vi "Cycle 4 Main Spin.vi"(0 "GEA2 Reference In":refnum<k24>, 1 "Basket Speeds (rpm)":u32[](array[numeric])=[125, 450, 700], 5 "GEA Inputs":T1={"Source"=228, "Destination"=35} {"Destination" format="%.0x"; "Source" format="%.0x"}, 7 "Standalone?":bool, 9 "Dwell Times (s)":dbl[](array[numeric])=[90.0, 30.0, 600.0], 11 "Error In":errorcluster, 12 "Basket Speed Tolerance (rpm)":u32=2) -> (4 "GEA2 Reference Out":refnum<k24>, 6 "Pass/Fail?":bool, 8 "Report Text":string, 15 "Error Out":errorcluster)   [LabVIEW 2016, in "2015 VA Washer.lvlib"]
uses:
  Projects/2015 VA Washer.lvlib
  C:/Automation/DLLs/PC Dot Net/GeaCommunication.dll
  Common/LabVIEW GEA2 Toolkit/LabVIEW_GEA2_Toolkit.lvlibp/type defs/Source_Destination.ctl
  Common/LabVIEW GEA2 Toolkit/LabVIEW_GEA2_Toolkit.lvlibp/type defs/ERD Read Data In.ctl
  Common/LabVIEW GEA2 Toolkit/LabVIEW_GEA2_Toolkit.lvlibp/type defs/Data Type.ctl
  Valew Common/type defs/Drive Cycle Engine Request State.ctl
  Common/LabVIEW GEA2 Toolkit/LabVIEW_GEA2_Toolkit.lvlibp
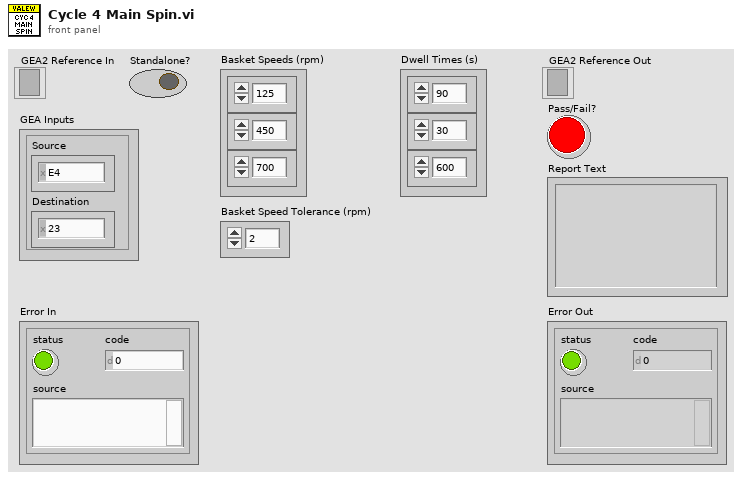
[diagram p1: front panel]
types:
  T1 = typedef "LabVIEW_GEA2_Toolkit.lvlibp/Source_Destination.ctl" = cluster{"Source":u8, "Destination":u8}
  T2 = typedef "2015 VA Washer.lvlib/Drive Cycle Engine Request State.ctl" = enum16{"Start", "Stop", "Pause", "Resume", "Select"}
  T3 = typedef "LabVIEW_GEA2_Toolkit.lvlibp/ERD Read Data In.ctl" = cluster{"ERD Number":u16, "Data Type":T4}
  T4 = typedef "LabVIEW_GEA2_Toolkit.lvlibp/Data Type.ctl" = enum16{"string", "boolean", "uint8_t", "uint16_t", "uint32_t", "uint64_t", "int8_t", "int16_t", "int32_t", "int64_t"}
  T5 = typedef "LabVIEW_GEA2_Toolkit.lvlibp/ERD Read Data Out.ctl" = cluster{"ERD Number":u16, "Data":string}
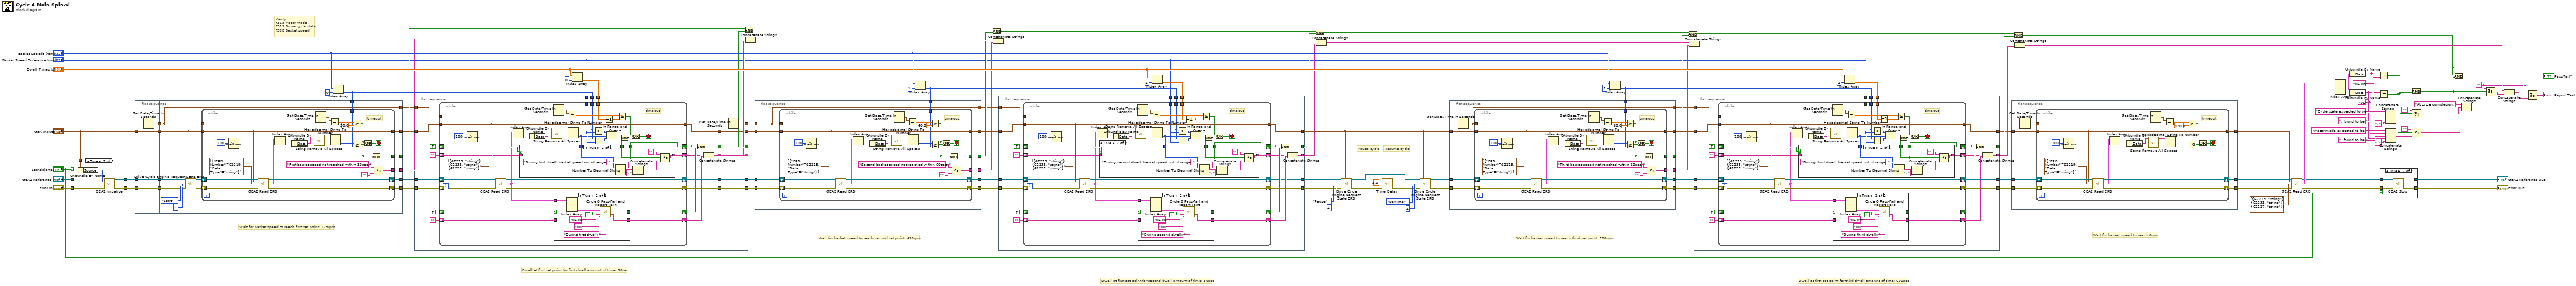
[diagram p0: block diagram]
diagram:
  w9 = ""
  w116 = "04 0B" ("y")
  w104 = "06" ("y")
  # "Wait for basket speed to reach 0rpm"
  # "Resume cycle"
  # "Pause cycle"
  # "Dwell at first set point for third dwell amount of time: 600sec"
  # "Wait for basket speed to reach third set point: 700rpm"
  # "Dwell at first set point for second dwell amount of time: 30sec"
  # "Wait for basket speed to reach second set point: 450rpm"
  # "Verify\nF313 Motor mode\nF319 Drive cycle state\nF30B Basket speed"
  # "Dwell at first set point for first dwell amount of time: 90sec"
  # "Wait for basket speed to reach first set point: 125rpm"
  n1 = case shown="True" "Standalone?" {
    tunnel: "GEA2 Reference In" -> [w123 _]
    tunnel: [w123 w128] -> w25
    tunnel: "Error In" -> [w122 w127]
    tunnel: [w122 w126] -> w26
    tunnel: "GEA Inputs" -> [_ w125]
    frame False {
    }
    frame True {
      n2 = Unbundle By Name(w125) -> ("Source"=w124:u8)
      n3 = call "GEA2 Initialize.vi"("Source Address"=w124, "error in"=w127) -> ("GEA2 Reference Out"=w128:refnum<k24>, "error out"=w126:errorcluster)  [unwired: 11 in, 1 out]
    }
  }
  n4 = flat-sequence {
    tunnel: "GEA Inputs" -> [w132]
    tunnel: [w132] -> w27
    tunnel: w26 -> [w129]
    tunnel: w25 -> [w130]
    tunnel: [w131] -> w24
    tunnel: [w130] -> w23
    tunnel: [w129] -> w22
    tunnel: [w146] -> w84
    tunnel: [w145] -> w85
    tunnel: [w144] -> w97
    tunnel: [w141] -> w50
    tunnel: [w142] -> w48
    tunnel: w66 -> [w143]
    tunnel: [w133] -> w30
    tunnel: w27 -> [w134]
    tunnel: w24 -> [w133]
    tunnel: w23 -> [w138]
    tunnel: w22 -> [w137]
    frame #0 {
      n5 = Get Date/Time In Seconds() -> (seconds since 1Jan1904=w131:timestamp)
    }
    frame #1 {
      n6 = call "Drive Cycle Engine Request State ERD.vi"("GEA2 Reference In"=w138, "GEA Inputs"=w134, "Cycle ID"=u8 4, "Drive Cycle Engine Request State"=Drive_Cycle_Engine_Request_State."Start", "Error In"=w137) -> ("GEA2 Reference Out"=w136:refnum<k24>, "Error Out"=w135:errorcluster)  [unwired: 9 in]
      n7 = while {
        shift-right: [w169] -> w146
        shift-left: w135 -> [w170]
        shift-right: [w167] -> w145
        shift-left: w136 -> [w168]
        tunnel: w134 -> [w165]
        tunnel: [w165] -> w144
        tunnel: w133 -> [w147]
        tunnel: w143 -> [w155]
        tunnel: [w150] -> w142
        tunnel: [w148] -> w141
        stop <- w162 stop-if-true
        # "timeout"
        n8 = Wait (ms)(milliseconds to wait=u32 100) -> ()  [unwired: 1 out]
        n9 = call "GEA2 Read ERD.vi"("GEA2 Reference In"=w168, "GEA Inputs"=w165, "Read ERD List"=T3[] [{"ERD Number"=62219, "Data Type"=enum."string"}], "Error In"=w170) -> ("GEA2 Reference Out"=w167:refnum<k24>, "ERD Data Out"=w154:T5[], "Error Out"=w169:errorcluster)  [unwired: 8 in, 1 out]
        n10 = Index Array(array=w154) -> (element=w166:T5)  [unwired: 1 in]
        n11 = Unbundle By Name(w166) -> ("Data"=w158:string)
        n12 = call "String Remove All Spaces.vi"("Input String"=w158) -> ("Spaces Removed"=w159:string)  [unwired: 13 in, 1 out]
        n13 = Get Date/Time In Seconds() -> (seconds since 1Jan1904=w163:timestamp)
        n14 = Subtract(x=w163, y=w147) -> (x-y=w164:dbl)
        n15 = Hexadecimal String To Number(string=w159) -> (number=w157:u32)  [unwired: 2 in, 1 out]
        n16 = Greater Or Equal?(x=w164, y=30.0) -> (x >= y?=w149:bool)
        n17 = Greater Or Equal?(x=w157, y=w155) -> (x >= y?=w153:bool)
        n18 = Or(x=w149, y=w153) -> (x .or. y?=w162:bool)
        n19 = Not(x=w149) -> (.not. x?=w148:bool)
        n20 = Select(t="First basket speed not reached within 30sec. ", s=w149, f="") -> (s? t:f=w150:string)
      }
    }
  }
  n21 = Index Array(array="Basket Speeds (rpm)", index=0) -> (element=w66:u32)
  n22 = flat-sequence {
    tunnel: w87 -> [w183]
    tunnel: w66 -> [w182]
    tunnel: "Basket Speed Tolerance (rpm)" -> [w181]
    tunnel: w84 -> [w188]
    tunnel: w97 -> [w189]
    tunnel: w85 -> [w190]
    tunnel: w30 -> [w171]
    tunnel: [w186] -> w5
    tunnel: [w185] -> w4
    tunnel: [w184] -> w3
    tunnel: [w175] -> w2
    tunnel: [w172] -> w1
    tunnel: [w245] -> w6
    tunnel: [w246] -> w47
    tunnel: [w247] -> w49
    tunnel: [w248] -> w81
    tunnel: [w249] -> w83
    tunnel: [w250] -> w82
    tunnel: w5 -> [w250]
    tunnel: w4 -> [w249]
    tunnel: w3 -> [w248]
    tunnel: w2 -> [w247]
    tunnel: w1 -> [w246]
    frame #0 {
      n23 = while {
        shift-right: [w222] -> w186
        shift-left: w188 -> [w223]
        shift-right: [w220] -> w185
        shift-left: w190 -> [w221]
        tunnel: w189 -> [w218]
        tunnel: [w218] -> w184
        tunnel: w171 -> [w216]
        shift-right: [w200] -> w176
        shift-left: TRUE -> [w202]
        tunnel: w183 -> [w192]
        tunnel: w182 -> [w207]
        tunnel: w181 -> [w206]
        shift-right: [w204] -> w173
        shift-left: "" -> [w201]
        shift-right: [w194] -> w177
        shift-left: TRUE -> [w197]
        shift-right: [w195] -> w174
        shift-left: "" -> [w196]
        stop <- w214 stop-if-true
        # "timeout"
        n24 = Wait (ms)(milliseconds to wait=u32 100) -> ()  [unwired: 1 out]
        n25 = call "GEA2 Read ERD.vi"("GEA2 Reference In"=w221, "GEA Inputs"=w218, "Read ERD List"=T3[] [{"ERD Number"=62219, "Data Type"=enum."string"}, {"ERD Number"=62233, "Data Type"=enum."string"}, {"ERD Number"=62227, "Data Type"=enum."string"}], "Error In"=w223) -> ("GEA2 Reference Out"=w220:refnum<k24>, "ERD Data Out"=w193:T5[], "Error Out"=w222:errorcluster)  [unwired: 8 in, 1 out]
        n26 = Index Array(array=w193) -> (element=w219:T5)  [unwired: 1 in]
        n27 = Unbundle By Name(w219) -> ("Data"=w210:string)
        n28 = call "String Remove All Spaces.vi"("Input String"=w210) -> ("Spaces Removed"=w211:string)  [unwired: 13 in, 1 out]
        n29 = Get Date/Time In Seconds() -> (seconds since 1Jan1904=w215:timestamp)
        n30 = case shown="True" w197 {
          selector: w197 -> [w224 _]
          tunnel: w196 -> [w225 _]
          tunnel: [w225 w233] -> w195
          tunnel: [w224 w234] -> w194
          tunnel: w193 -> [_ w232]
          frame False {
          }
          frame True {
            n31 = Index Array(array=w232) -> (element #2=w230:T5, element #3=w229:T5)  [unwired: 3 in, 1 out]
            n32 = call "Cycle 0 Pass-Fail and Report Text.vi"("Drive Cycle State"=w230, "Motor Mode"=w229, "Previous Pass/Fail"=TRUE, "Cycle State Expected"="04 06", "Motor Mode Expected"="00", "Header"="During first dwell: ") -> ("Pass/Fail?"=w234:bool, "Report Text"=w233:string)  [unwired: 8 in]
          }
        }
        n33 = Subtract(x=w215, y=w216) -> (x-y=w217:dbl)
        n34 = Hexadecimal String To Number(string=w211) -> (number=w205:u32)  [unwired: 2 in, 1 out]
        n35 = Add(x=w207, y=w206) -> (x+y=w209:u32)
        n36 = Subtract(x=w207, y=w206) -> (x-y=w208:u32)
        n37 = Decrement(x=w192) -> (x-1=w191:dbl)
        n38 = In Range and Coerce(upper limit=w209, x=w205, lower limit=w208) -> (In Range?=w203:bool)  [unwired: 1 out]
        n39 = case shown="True" w202 {
          selector: w202 -> [w235 _]
          tunnel: w205 -> [_ w242]
          tunnel: [w236 w239] -> w204
          tunnel: w203 -> [_ w238]
          tunnel: w201 -> [w236 _]
          tunnel: [w235 w238] -> w200
          frame False {
          }
          frame True {
            n40 = Number To Decimal String(number=w242) -> (decimal integer string=w241:string)  [unwired: 1 in]
            n41 = Concatenate Strings("During first dwell, basket speed out of range: " ("string"), w241, ". " ("string")) -> (w240:string)
            n42 = Select(t="", s=w238, f=w240) -> (s? t:f=w239:string)
          }
        }
        n43 = Greater Or Equal?(x=w217, y=w191) -> (x >= y?=w198:bool)
        n44 = Not(x=w203) -> (.not. x?=w199:bool)
        n45 = Or(x=w198, y=w199) -> (x .or. y?=w214:bool)
      }
      n46 = And(x=w176, y=w177) -> (x .and. y?=w175:bool)
      n47 = Concatenate Strings(w173, w174) -> (w172:string)
    }
    frame #1 {
      n48 = Get Date/Time In Seconds() -> (seconds since 1Jan1904=w245:timestamp)
    }
  }
  n49 = Index Array(array="Dwell Times (s)", index=0) -> (element=w87:dbl)
  n50 = And(x=w50, y=w49) -> (x .and. y?=w46:bool)
  n51 = Concatenate Strings(w48, w47) -> (w45:string)
  n52 = flat-sequence {
    tunnel: [w257] -> w79
    tunnel: [w256] -> w78
    tunnel: [w255] -> w77
    tunnel: [w252] -> w43
    tunnel: [w253] -> w44
    tunnel: w76 -> [w254]
    tunnel: w82 -> [w258]
    tunnel: w81 -> [w259]
    tunnel: w83 -> [w260]
    tunnel: [w251] -> w29
    tunnel: w6 -> [w251]
    frame #0 {
      n53 = while {
        shift-right: [w283] -> w257
        shift-left: w258 -> [w284]
        shift-right: [w281] -> w256
        shift-left: w260 -> [w282]
        tunnel: w259 -> [w279]
        tunnel: [w279] -> w255
        tunnel: w251 -> [w261]
        tunnel: w254 -> [w269]
        tunnel: [w264] -> w253
        tunnel: [w262] -> w252
        stop <- w276 stop-if-true
        # "timeout"
        n54 = Wait (ms)(milliseconds to wait=u32 100) -> ()  [unwired: 1 out]
        n55 = call "GEA2 Read ERD.vi"("GEA2 Reference In"=w282, "GEA Inputs"=w279, "Read ERD List"=T3[] [{"ERD Number"=62219, "Data Type"=enum."string"}], "Error In"=w284) -> ("GEA2 Reference Out"=w281:refnum<k24>, "ERD Data Out"=w268:T5[], "Error Out"=w283:errorcluster)  [unwired: 8 in, 1 out]
        n56 = Index Array(array=w268) -> (element=w280:T5)  [unwired: 1 in]
        n57 = Unbundle By Name(w280) -> ("Data"=w272:string)
        n58 = call "String Remove All Spaces.vi"("Input String"=w272) -> ("Spaces Removed"=w273:string)  [unwired: 13 in, 1 out]
        n59 = Get Date/Time In Seconds() -> (seconds since 1Jan1904=w277:timestamp)
        n60 = Subtract(x=w277, y=w261) -> (x-y=w278:dbl)
        n61 = Hexadecimal String To Number(string=w273) -> (number=w271:u32)  [unwired: 2 in, 1 out]
        n62 = Greater Or Equal?(x=w278, y=60.0) -> (x >= y?=w263:bool)
        n63 = Greater Or Equal?(x=w271, y=w269) -> (x >= y?=w267:bool)
        n64 = Or(x=w263, y=w267) -> (x .or. y?=w276:bool)
        n65 = Not(x=w263) -> (.not. x?=w262:bool)
        n66 = Select(t="Second basket speed not reached within 60sec. ", s=w263, f="") -> (s? t:f=w264:string)
      }
    }
  }
  n67 = Index Array(array="Basket Speeds (rpm)", index=1) -> (element=w76:u32)
  n68 = And(x=w46, y=w43) -> (x .and. y?=w40:bool)
  n69 = Concatenate Strings(w45, w44) -> (w41:string)
  n70 = flat-sequence {
    tunnel: [w300] -> w60
    tunnel: [w299] -> w51
    tunnel: [w290] -> w39
    tunnel: [w287] -> w42
    tunnel: w74 -> [w298]
    tunnel: w76 -> [w297]
    tunnel: "Basket Speed Tolerance (rpm)" -> [w296]
    tunnel: w79 -> [w302]
    tunnel: w77 -> [w303]
    tunnel: w78 -> [w304]
    tunnel: [w286] -> w61
    tunnel: w29 -> [w285]
    frame #0 {
      n71 = while {
        shift-right: [w336] -> w300
        shift-left: w302 -> [w337]
        shift-right: [w334] -> w286
        shift-left: w304 -> [w335]
        tunnel: w303 -> [w332]
        tunnel: [w332] -> w299
        tunnel: w285 -> [w330]
        shift-right: [w314] -> w291
        shift-left: TRUE -> [w316]
        tunnel: w298 -> [w306]
        tunnel: w297 -> [w321]
        tunnel: w296 -> [w320]
        shift-right: [w318] -> w288
        shift-left: "" -> [w315]
        shift-right: [w308] -> w292
        shift-left: TRUE -> [w311]
        shift-right: [w309] -> w289
        shift-left: "" -> [w310]
        stop <- w328 stop-if-true
        # "timeout"
        n72 = Wait (ms)(milliseconds to wait=u32 100) -> ()  [unwired: 1 out]
        n73 = call "GEA2 Read ERD.vi"("GEA2 Reference In"=w335, "GEA Inputs"=w332, "Read ERD List"=T3[] [{"ERD Number"=62219, "Data Type"=enum."string"}, {"ERD Number"=62233, "Data Type"=enum."string"}, {"ERD Number"=62227, "Data Type"=enum."string"}], "Error In"=w337) -> ("GEA2 Reference Out"=w334:refnum<k24>, "ERD Data Out"=w307:T5[], "Error Out"=w336:errorcluster)  [unwired: 8 in, 1 out]
        n74 = Index Array(array=w307) -> (element=w333:T5)  [unwired: 1 in]
        n75 = Unbundle By Name(w333) -> ("Data"=w324:string)
        n76 = call "String Remove All Spaces.vi"("Input String"=w324) -> ("Spaces Removed"=w325:string)  [unwired: 13 in, 1 out]
        n77 = Get Date/Time In Seconds() -> (seconds since 1Jan1904=w329:timestamp)
        n78 = case shown="True" w311 {
          selector: w311 -> [w338 _]
          tunnel: w310 -> [w339 _]
          tunnel: [w339 w347] -> w309
          tunnel: [w338 w348] -> w308
          tunnel: w307 -> [_ w346]
          frame False {
          }
          frame True {
            n79 = Index Array(array=w346) -> (element #2=w344:T5, element #3=w343:T5)  [unwired: 3 in, 1 out]
            n80 = call "Cycle 0 Pass-Fail and Report Text.vi"("Drive Cycle State"=w344, "Motor Mode"=w343, "Previous Pass/Fail"=TRUE, "Cycle State Expected"="04 06", "Motor Mode Expected"="00", "Header"="During second dwell: ") -> ("Pass/Fail?"=w348:bool, "Report Text"=w347:string)  [unwired: 8 in]
          }
        }
        n81 = Subtract(x=w329, y=w330) -> (x-y=w331:dbl)
        n82 = Hexadecimal String To Number(string=w325) -> (number=w319:u32)  [unwired: 2 in, 1 out]
        n83 = Add(x=w321, y=w320) -> (x+y=w323:u32)
        n84 = Subtract(x=w321, y=w320) -> (x-y=w322:u32)
        n85 = Decrement(x=w306) -> (x-1=w305:dbl)
        n86 = In Range and Coerce(upper limit=w323, x=w319, lower limit=w322) -> (In Range?=w317:bool)  [unwired: 1 out]
        n87 = case shown="True" w316 {
          selector: w316 -> [w349 _]
          tunnel: w319 -> [_ w356]
          tunnel: [w350 w353] -> w318
          tunnel: w317 -> [_ w352]
          tunnel: w315 -> [w350 _]
          tunnel: [w349 w352] -> w314
          frame False {
          }
          frame True {
            n88 = Number To Decimal String(number=w356) -> (decimal integer string=w355:string)  [unwired: 1 in]
            n89 = Concatenate Strings("During second dwell, basket speed out of range: " ("string"), w355, ". " ("string")) -> (w354:string)
            n90 = Select(t="", s=w352, f=w354) -> (s? t:f=w353:string)
          }
        }
        n91 = Greater Or Equal?(x=w331, y=w305) -> (x >= y?=w312:bool)
        n92 = Not(x=w317) -> (.not. x?=w313:bool)
        n93 = Or(x=w312, y=w313) -> (x .or. y?=w328:bool)
      }
      n94 = And(x=w291, y=w292) -> (x .and. y?=w290:bool)
      n95 = Concatenate Strings(w288, w289) -> (w287:string)
    }
  }
  n96 = Index Array(array="Dwell Times (s)", index=1) -> (element=w74:dbl)
  n97 = And(x=w40, y=w39) -> (x .and. y?=w38:bool)
  n98 = Concatenate Strings(w41, w42) -> (w37:string)
  n99 = call "Drive Cycle Engine Request State ERD.vi"("GEA2 Reference In"=w61, "GEA Inputs"=w51, "Cycle ID"=u8 4, "Drive Cycle Engine Request State"=Drive_Cycle_Engine_Request_State."Pause", "Error In"=w60) -> ("GEA2 Reference Out"=w54:refnum<k24>, "Error Out"=w59:errorcluster)  [unwired: 9 in]
  n100 = call "Time Delay"("error in (no error)"=w59, "Delay Time (s)"=3.0) -> ("error out"=w55:errorcluster)  [unwired: 9 in]
  n101 = call "Drive Cycle Engine Request State ERD.vi"("GEA2 Reference In"=w54, "GEA Inputs"=w51, "Cycle ID"=u8 4, "Drive Cycle Engine Request State"=Drive_Cycle_Engine_Request_State."Resume", "Error In"=w55) -> ("GEA2 Reference Out"=w52:refnum<k24>, "Error Out"=w56:errorcluster)  [unwired: 9 in]
  n102 = flat-sequence {
    tunnel: [w365] -> w72
    tunnel: [w364] -> w71
    tunnel: [w363] -> w70
    tunnel: [w360] -> w35
    tunnel: [w361] -> w36
    tunnel: w69 -> [w362]
    tunnel: w56 -> [w366]
    tunnel: w51 -> [w367]
    tunnel: w52 -> [w368]
    tunnel: [w359] -> w28
    frame #0 {
      n103 = Get Date/Time In Seconds() -> (seconds since 1Jan1904=w359:timestamp)
      n104 = while {
        shift-right: [w391] -> w365
        shift-left: w366 -> [w392]
        shift-right: [w389] -> w364
        shift-left: w368 -> [w390]
        tunnel: w367 -> [w387]
        tunnel: [w387] -> w363
        tunnel: w359 -> [w369]
        tunnel: w362 -> [w377]
        tunnel: [w372] -> w361
        tunnel: [w370] -> w360
        stop <- w384 stop-if-true
        # "timeout"
        n105 = Wait (ms)(milliseconds to wait=u32 100) -> ()  [unwired: 1 out]
        n106 = call "GEA2 Read ERD.vi"("GEA2 Reference In"=w390, "GEA Inputs"=w387, "Read ERD List"=T3[] [{"ERD Number"=62219, "Data Type"=enum."string"}], "Error In"=w392) -> ("GEA2 Reference Out"=w389:refnum<k24>, "ERD Data Out"=w376:T5[], "Error Out"=w391:errorcluster)  [unwired: 8 in, 1 out]
        n107 = Index Array(array=w376) -> (element=w388:T5)  [unwired: 1 in]
        n108 = Unbundle By Name(w388) -> ("Data"=w380:string)
        n109 = call "String Remove All Spaces.vi"("Input String"=w380) -> ("Spaces Removed"=w381:string)  [unwired: 13 in, 1 out]
        n110 = Get Date/Time In Seconds() -> (seconds since 1Jan1904=w385:timestamp)
        n111 = Subtract(x=w385, y=w369) -> (x-y=w386:dbl)
        n112 = Hexadecimal String To Number(string=w381) -> (number=w379:u32)  [unwired: 2 in, 1 out]
        n113 = Greater Or Equal?(x=w386, y=60.0) -> (x >= y?=w371:bool)
        n114 = Greater Or Equal?(x=w379, y=w377) -> (x >= y?=w375:bool)
        n115 = Or(x=w371, y=w375) -> (x .or. y?=w384:bool)
        n116 = Not(x=w371) -> (.not. x?=w370:bool)
        n117 = Select(t="Third basket speed not reached within 60sec. ", s=w371, f="") -> (s? t:f=w372:string)
      }
    }
  }
  n118 = Index Array(array="Basket Speeds (rpm)", index=2) -> (element=w69:u32)
  n119 = And(x=w38, y=w35) -> (x .and. y?=w34:bool)
  n120 = Concatenate Strings(w37, w36) -> (w33:string)
  n121 = flat-sequence {
    tunnel: [w408] -> w20
    tunnel: [w407] -> w21
    tunnel: [w406] -> w19
    tunnel: [w397] -> w31
    tunnel: [w394] -> w32
    tunnel: w67 -> [w405]
    tunnel: w69 -> [w404]
    tunnel: "Basket Speed Tolerance (rpm)" -> [w403]
    tunnel: w72 -> [w410]
    tunnel: w70 -> [w411]
    tunnel: w71 -> [w412]
    tunnel: w28 -> [w393]
    frame #0 {
      n122 = while {
        shift-right: [w444] -> w408
        shift-left: w410 -> [w445]
        shift-right: [w442] -> w407
        shift-left: w412 -> [w443]
        tunnel: w411 -> [w440]
        tunnel: [w440] -> w406
        tunnel: w393 -> [w438]
        shift-right: [w422] -> w398
        shift-left: TRUE -> [w424]
        tunnel: w405 -> [w414]
        tunnel: w404 -> [w429]
        tunnel: w403 -> [w428]
        shift-right: [w426] -> w395
        shift-left: "" -> [w423]
        shift-right: [w416] -> w399
        shift-left: TRUE -> [w419]
        shift-right: [w417] -> w396
        shift-left: "" -> [w418]
        stop <- w436 stop-if-true
        # "timeout"
        n123 = Wait (ms)(milliseconds to wait=u32 100) -> ()  [unwired: 1 out]
        n124 = call "GEA2 Read ERD.vi"("GEA2 Reference In"=w443, "GEA Inputs"=w440, "Read ERD List"=T3[] [{"ERD Number"=62219, "Data Type"=enum."string"}, {"ERD Number"=62233, "Data Type"=enum."string"}, {"ERD Number"=62227, "Data Type"=enum."string"}], "Error In"=w445) -> ("GEA2 Reference Out"=w442:refnum<k24>, "ERD Data Out"=w415:T5[], "Error Out"=w444:errorcluster)  [unwired: 8 in, 1 out]
        n125 = Index Array(array=w415) -> (element=w441:T5)  [unwired: 1 in]
        n126 = Unbundle By Name(w441) -> ("Data"=w432:string)
        n127 = call "String Remove All Spaces.vi"("Input String"=w432) -> ("Spaces Removed"=w433:string)  [unwired: 13 in, 1 out]
        n128 = Get Date/Time In Seconds() -> (seconds since 1Jan1904=w437:timestamp)
        n129 = case shown="True" w419 {
          selector: w419 -> [w446 _]
          tunnel: w418 -> [w447 _]
          tunnel: [w447 w455] -> w417
          tunnel: [w446 w456] -> w416
          tunnel: w415 -> [_ w454]
          frame False {
          }
          frame True {
            n130 = Index Array(array=w454) -> (element #2=w452:T5, element #3=w451:T5)  [unwired: 3 in, 1 out]
            n131 = call "Cycle 0 Pass-Fail and Report Text.vi"("Drive Cycle State"=w452, "Motor Mode"=w451, "Previous Pass/Fail"=TRUE, "Cycle State Expected"="04 09", "Motor Mode Expected"="00", "Header"="During third dwell: ") -> ("Pass/Fail?"=w456:bool, "Report Text"=w455:string)  [unwired: 8 in]
          }
        }
        n132 = Subtract(x=w437, y=w438) -> (x-y=w439:dbl)
        n133 = Hexadecimal String To Number(string=w433) -> (number=w427:u32)  [unwired: 2 in, 1 out]
        n134 = Add(x=w429, y=w428) -> (x+y=w431:u32)
        n135 = Subtract(x=w429, y=w428) -> (x-y=w430:u32)
        n136 = Decrement(x=w414) -> (x-1=w413:dbl)
        n137 = In Range and Coerce(upper limit=w431, x=w427, lower limit=w430) -> (In Range?=w425:bool)  [unwired: 1 out]
        n138 = case shown="True" w424 {
          selector: w424 -> [w457 _]
          tunnel: w427 -> [_ w464]
          tunnel: [w458 w461] -> w426
          tunnel: w425 -> [_ w460]
          tunnel: w423 -> [w458 _]
          tunnel: [w457 w460] -> w422
          frame False {
          }
          frame True {
            n139 = Number To Decimal String(number=w464) -> (decimal integer string=w463:string)  [unwired: 1 in]
            n140 = Concatenate Strings("During third dwell, basket speed out of range: " ("string"), w463, ". " ("string")) -> (w462:string)
            n141 = Select(t="", s=w460, f=w462) -> (s? t:f=w461:string)
          }
        }
        n142 = Greater Or Equal?(x=w439, y=w413) -> (x >= y?=w420:bool)
        n143 = Not(x=w425) -> (.not. x?=w421:bool)
        n144 = Or(x=w420, y=w421) -> (x .or. y?=w436:bool)
      }
      n145 = And(x=w398, y=w399) -> (x .and. y?=w397:bool)
      n146 = Concatenate Strings(w395, w396) -> (w394:string)
    }
  }
  n147 = Index Array(array="Dwell Times (s)", index=2) -> (element=w67:dbl)
  n148 = flat-sequence {
    tunnel: [w469] -> w16
    tunnel: [w468] -> w17
    tunnel: [w467] -> w18
    tunnel: w20 -> [w471]
    tunnel: w19 -> [w472]
    tunnel: w21 -> [w473]
    frame #0 {
      n149 = Get Date/Time In Seconds() -> (seconds since 1Jan1904=w470:timestamp)
      n150 = while {
        shift-right: [w491] -> w469
        shift-left: w471 -> [w492]
        shift-right: [w489] -> w468
        shift-left: w473 -> [w490]
        tunnel: w472 -> [w487]
        tunnel: [w487] -> w467
        tunnel: w470 -> [w474]
        stop <- w484 stop-if-true
        # "timeout"
        n151 = Wait (ms)(milliseconds to wait=u32 100) -> ()  [unwired: 1 out]
        n152 = call "GEA2 Read ERD.vi"("GEA2 Reference In"=w490, "GEA Inputs"=w487, "Read ERD List"=T3[] [{"ERD Number"=62219, "Data Type"=enum."string"}], "Error In"=w492) -> ("GEA2 Reference Out"=w489:refnum<k24>, "ERD Data Out"=w477:T5[], "Error Out"=w491:errorcluster)  [unwired: 8 in, 1 out]
        n153 = Index Array(array=w477) -> (element=w488:T5)  [unwired: 1 in]
        n154 = Unbundle By Name(w488) -> ("Data"=w480:string)
        n155 = call "String Remove All Spaces.vi"("Input String"=w480) -> ("Spaces Removed"=w481:string)  [unwired: 13 in, 1 out]
        n156 = Get Date/Time In Seconds() -> (seconds since 1Jan1904=w485:timestamp)
        n157 = Subtract(x=w485, y=w474) -> (x-y=w486:dbl)
        n158 = Hexadecimal String To Number(string=w481) -> (number=w479:u32)  [unwired: 2 in, 1 out]
        n159 = Greater Or Equal?(x=w486, y=120.0) -> (x >= y?=w475:bool)
        n160 = Equal To 0?(x=w479) -> (x = 0?=w476:bool)
        n161 = Or(x=w475, y=w476) -> (x .or. y?=w484:bool)
      }
    }
  }
  n162 = And(x=w34, y=w31) -> (x .and. y?=w10:bool)
  n163 = Concatenate Strings(w33, w32) -> (w12:string)
  n164 = call "GEA2 Read ERD.vi"("GEA2 Reference In"=w17, "GEA Inputs"=w18, "Read ERD List"=T3[] [{"ERD Number"=62219, "Data Type"=enum."string"}, {"ERD Number"=62233, "Data Type"=enum."string"}, {"ERD Number"=62227, "Data Type"=enum."string"}], "Error In"=w16) -> ("GEA2 Reference Out"=w91:refnum<k24>, "ERD Data Out"=w118:T5[], "Error Out"=w93:errorcluster)  [unwired: 8 in, 1 out]
  n165 = Index Array(array=w118) -> (element #2=w121:T5, element #3=w120:T5)  [unwired: 3 in, 1 out]
  n166 = Unbundle By Name(w121) -> ("Data"=w114:string)
  n167 = Unbundle By Name(w120) -> ("Data"=w102:string)
  n168 = Equal?(x=w114, y=w116) -> (x = y?=w111:bool)
  n169 = Equal?(x=w102, y=w104) -> (x = y?=w110:bool)
  n170 = case shown="True" "Standalone?" {
    tunnel: [w493 w497] -> w94
    tunnel: w93 -> [w493 w496]
    tunnel: w91 -> [w494 w495]
    tunnel: [w494 _] -> w90
    frame False {
    }
    frame True {
      n171 = call "GEA2 Stop.vi"("GEA2 Reference In"=w495, "Error In"=w496) -> ("Error Out"=w497:errorcluster)  [unwired: 13 in]
    }
  }
  "GEA2 Reference Out" <- w90
  "Error Out" <- w94
  n172 = Concatenate Strings("Cycle state expected to be " ("string"), w116, ", found to be " ("string"), w114, ". " ("string")) -> (w112:string)
  n173 = Concatenate Strings("Motor mode expected to be " ("string"), w104, ", found to be " ("string"), w102, ". " ("string")) -> (w107:string)
  n174 = And(x=w110, y=w111) -> (x .and. y?=w14:bool)
  n175 = Select(t="", s=w111, f=w112) -> (s? t:f=w100:string)
  n176 = Select(t="", s=w110, f=w107) -> (s? t:f=w99:string)
  n177 = And(x=w10, y=w14) -> (x .and. y?=→"Pass/Fail?":bool)
  n178 = Concatenate Strings("At cycle completion: " ("string"), w100, w99) -> (w106:string)
  n179 = Select(t=w9, s=w14, f=w106) -> (s? t:f=w11:string)
  n180 = Concatenate Strings(w12, w11) -> (w8:string)
  n181 = Select(t=w9, s=w10, f=w8) -> (s? t:f=→"Report Text":string)
